vi "Close_Test.vi"(8 "error in (no error)":errorcluster caption="entrée d'erreur (pas d'erreur)", 11 "Test (Default) en entrée":refnum<class "Sequencer_With_Database.lvclass">) -> (0 "error out":errorcluster caption="sortie d'erreur", 3 "Test (Default) en sortie":refnum<class "Sequencer_With_Database.lvclass">)   [LabVIEW 2020, in "Library Core.lvlib" / "Sequencer_With_Database.lvclass"]
uses:
  Sequencer_With_Database.lvclass
  Sequencer (Default)/Sequencer (Default).lvclass
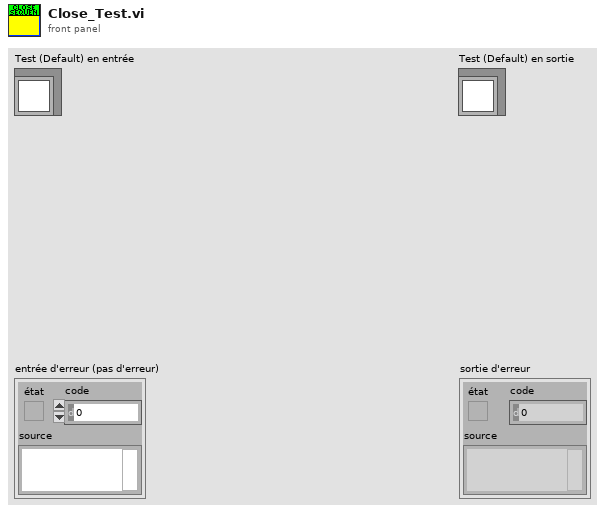
[diagram p1: front panel]
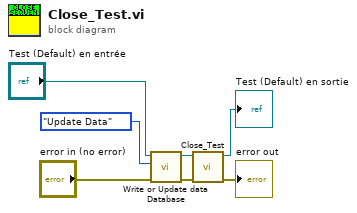
[diagram p0: block diagram]
diagram:
  n1 = call-dynamic "Write or Update data Database.vi"("error in (no error)"="error in (no error)", "Function"=enum16{"Set Data", "Update Data"}."Update Data", "Sequencer IN"="Test (Default) en entrée") -> ("error out"=w1:errorcluster, "Sequencer Out"=w5:refnum<class "Sequencer_With_Database.lvclass">)  [unwired: 7 in]
  n2 = call-parent "Close_Test.vi"("error in (no error)"=w1, "Test (Default) en entrée"=w5) -> ("error out"=→"error out":errorcluster, "Test (Default) en sortie"=→"Test (Default) en sortie":refnum<class "Sequencer_With_Database.lvclass">)  [unwired: 8 in]
